vi "Map Panes.vi"(8 "Error In":errorcluster, 10 "Control Refs":refnum<vi>[](array[refnum]), 11 "UI Panes In":T1) -> (0 "Error Out":errorcluster, 3 "UI Panes Out":T1)   [LabVIEW 2021, in "Appearance Actor.lvlib" / "Appearance Actor.lvclass"]
uses:
  Appearance Actor.lvclass
  Typedefs/UI Panes--map.ctl
  Typedefs/Element Panes--map.ctl
  Typedefs/Panes--map.ctl
  <vilib>/Utility/miscctls.llb/LVMapReplaceAction.ctl
  <vilib>/regexp/Match Regular Expression.xnode
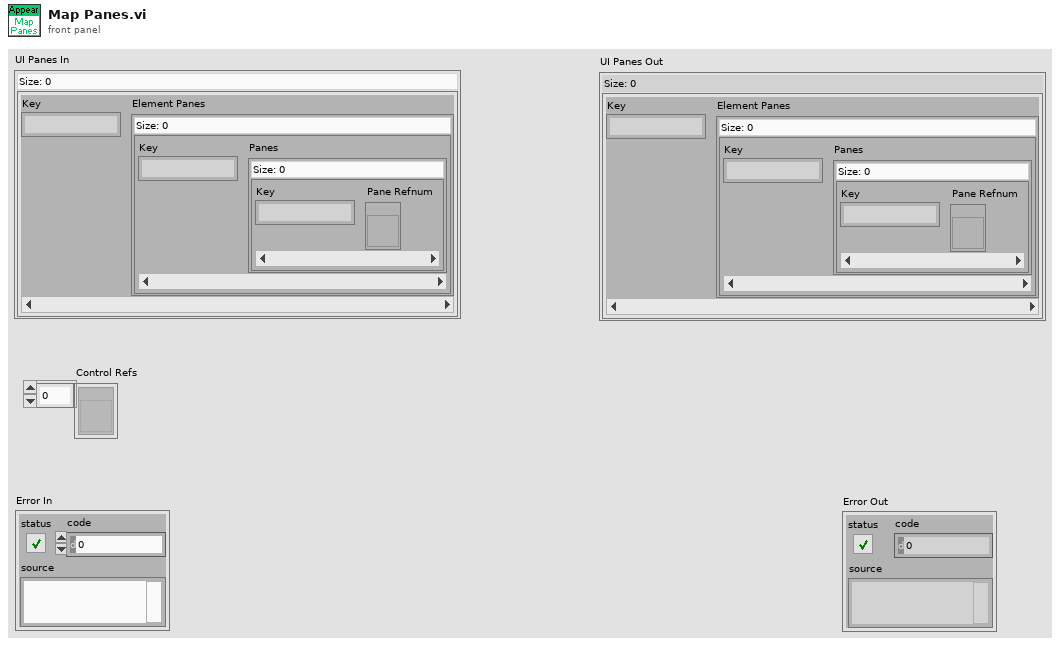
[diagram p1: front panel]
types:
  T1 = typedef "Appearance Actor.lvlib/Appearance Actor.lvclass/UI Panes--map.ctl" = map{string, T2}
  T2 = typedef "Appearance Actor.lvlib/Appearance Actor.lvclass/Element Panes--map.ctl" = map{string, T3}
  T3 = typedef "Appearance Actor.lvlib/Appearance Actor.lvclass/Panes--map.ctl" = map{string, refnum<vi>}
  T4 = typedef "LVMapReplaceAction.ctl" = enum32{"Modify Entry only if found", "Add or Modify Entry", "Delete Entry"}
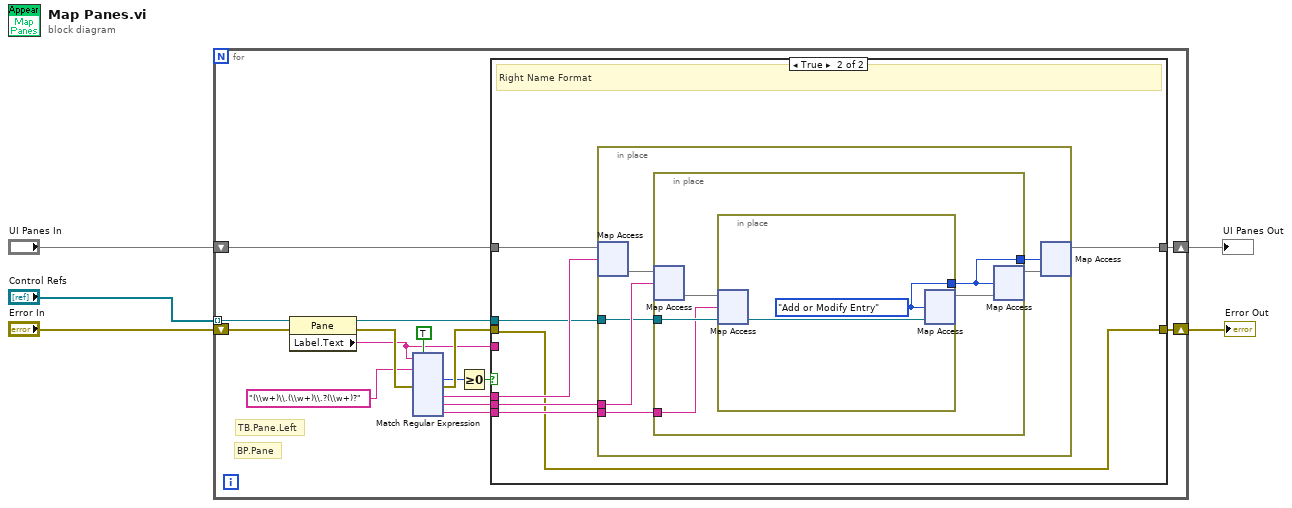
[diagram p0: block diagram]
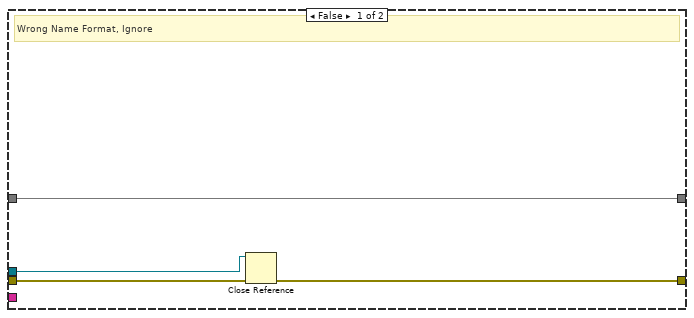
[diagram p2: hidden frame]
diagram:
  n1 = for {
    shift-right: [w11] -> w1
    shift-left: "UI Panes In" -> [w16]
    shift-right: [w15] -> w5
    shift-left: "Error In" -> [w20]
    tunnel: "Control Refs" -> [w21] mode=indexing
    # "BP.Pane"
    # "TB.Pane.Left"
    n2 = property class="Pane"(reference=w21, error in=w20) -> (reference out=w10:refnum<vi>, error out=w19:errorcluster, "Label.Text"=w12:string)
    n3 = xnode "Match Regular Expression"("input string"=w12, "regular expression"="(\\w+)\\.(\\w+)\\.?(\\w+)?", "error in"=w19, "ignore case? (F)"=TRUE) -> ("offset past match"=w9:i32, "error out"=w14:errorcluster, "submatch 1"=w7:string, "submatch 2"=w6:string, "submatch 3"=w13:string)  [unwired: 2 in, 3 out]
    n4 = Greater Or Equal To 0?(x=w9) -> (x >= 0?=w8:bool)
    n5 = case shown="True" w8 {
      tunnel: w16 -> [w25 w32]
      tunnel: w7 -> [_ w31]
      tunnel: [w22 w26] -> w15
      tunnel: w14 -> [w23 w26]
      tunnel: w6 -> [_ w29]
      tunnel: w13 -> [_ w28]
      tunnel: w12 -> [_ _]
      tunnel: [w25 w27] -> w11
      tunnel: w10 -> [w24 w30]
      frame False {
        # "Wrong Name Format, Ignore"
        n6 = Close Reference(reference=w24, error in (no error)=w23) -> (error out=w22:errorcluster)
      }
      frame True {
        # "Right Name Format"
        n7 = in-place {
          in-place-border: w29 -> [w37]
          in-place-border: w30 -> [w36]
          in-place-border: w28 -> [w34]
          n8 = in-place-map #1(w32, w31) -> (w38:T2)  [unwired: 1 in, 1 out]
          n9 = in-place {
            in-place-border: w36 -> [w42]
            in-place-border: [w41] -> w35
            in-place-border: w34 -> [w40]
            n10 = in-place-map #2(w38, w37) -> (w43:T3)  [unwired: 1 in, 1 out]
            n11 = in-place {
              in-place-border: [w44] -> w41
              w44 = LVMapReplaceAction."Add or Modify Entry" ("action")
              n12 = in-place-map #3(w43, w40, w42) -> (w45:refnum<vi>)  [unwired: 1 out]
              n13 = in-place-map #3(w45, w44) -> (w39:T3)  [unwired: 2 out]
            }
            n14 = in-place-map #2(w39, w41) -> (w33:T2)  [unwired: 2 out]
          }
          n15 = in-place-map #1(w33, w35) -> (w27:T1)  [unwired: 2 out]
        }
      }
    }
  }
  "Error Out" <- w5
  "UI Panes Out" <- w1
